vi "Read Logging Path.vi"(8 "error in (no error)":errorcluster, 11 "DemoClass in":refnum<class "DemoClass.lvclass">) -> (0 "error out":errorcluster, 2 "Logging Path":path, 3 "DemoClass out":refnum<class "DemoClass.lvclass">)   [LabVIEW 2020, in "VolatusScratch.lvlib" / "DemoClass.lvclass"]
uses:
  DemoClass.lvclass
  DemoClass.lvclass/DemoClass.ctl
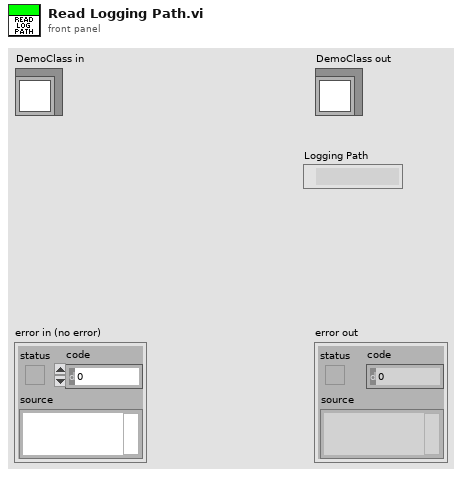
[diagram p1: front panel]
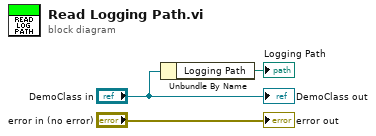
[diagram p0: block diagram]
diagram:
  n1 = Unbundle By Name("DemoClass in") -> ("Logging Path"=→"Logging Path":path)
  "error out" <- "error in (no error)"
  "DemoClass out" <- "DemoClass in"
